vi "Handling Incoming Bytes Tests.vi"(8 "error in (no error)":errorcluster) -> (0 "error out":errorcluster)   [LabVIEW 2013]
uses:
  source/Control Packets/ControlPacket/Control Packet Type -- enum.ctl
  source/Control Packets/CONNACK/Connect Return Code -- enum.ctl
  source/Control Packets/SUBSCRIBE/Topic Subscription -- cluster.ctl
  source/Control Packets/ControlPacket/QualityOfService -- enum.ctl
  source/Control Packets/SUBACK/Subscription Success Code.ctl
  source/Control Packets/CONNECT/ConnectPayload -- cluster.ctl
  source/Control Packets/ControlPacket/ControlPacket.lvclass
  source/Control Packets/CONNECT/CONNECT.lvclass
  source/Control Packets/CONNACK/CONNACK.lvclass
  source/Control Packets/PINGREQ/PINGREQ.lvclass
  source/Control Packets/PINGRESP/PINGRESP.lvclass
  source/Control Packets/PUBACK/PUBACK.lvclass
  source/Control Packets/PUBCOMP/PUBCOMP.lvclass
  source/Control Packets/PUBLISH/PUBLISH.lvclass
  source/Control Packets/PUBREC/PUBREC.lvclass
  source/Control Packets/PUBREL/PUBREL.lvclass
  source/Control Packets/SUBACK/SUBACK.lvclass
  source/Control Packets/SUBSCRIBE/SUBSCRIBE.lvclass
  source/Control Packets/UNSUBACK/UNSUBACK.lvclass
  source/Control Packets/UNSUBSCRIBE/UNSUBSCRIBE.lvclass
  source/Control Packets/DISCONNECT/DISCONNECT.lvclass
  <vilib>/addons/_JKI Toolkits/Caraya/classes/Test/Test.lvclass
panel:
  out "Packets Encoded":T1[](array[typedef])
  out "Packets decoded":T1[](array[typedef])
  out "Split message in single byte transmissions":bool
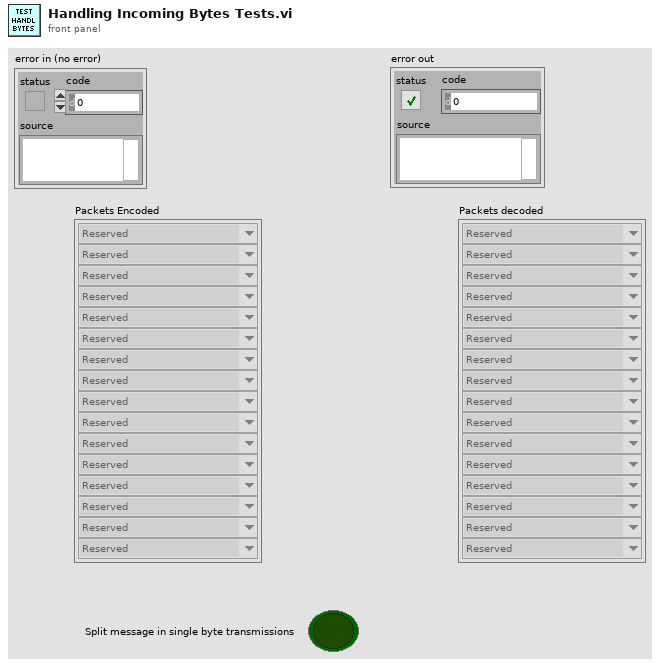
[diagram p1: front panel]
types:
  T1 = typedef "MQTT_Control_Packets.lvlib/ControlPacket.lvclass/Control Packet Type -- enum.ctl" = enum16{"Reserved", "CONNECT", "CONNACK", "PUBLISH", "PUBACK", "PUBREC", "PUBREL", "PUBCOMP", "SUBSCRIBE", "SUBACK", "UNSUBSCRIBE", "UNSUBACK", "PINGREQ", "PINGRESP", "DISCONNECT", "AUTH"}
  T2 = typedef "MQTT_Control_Packets.lvlib/CONNECT.lvclass/ConnectPayload -- cluster.ctl" = cluster{"Will Topic":string, "Will Message":string, "Username":string, "Password":string}
  T3 = typedef "MQTT_Control_Packets.lvlib/SUBACK.lvclass/Subscription Success Code.ctl" = cluster{"Subscription Failure":bool, "QoS":T4}
  T4 = typedef "MQTT_Control_Packets.lvlib/ControlPacket.lvclass/QualityOfService -- enum.ctl" = enum16{"0 (At Most Once)", "1 (At Least Once)", "2 (Exactly Once)"}
  T5 = typedef "MQTT_Control_Packets.lvlib/SUBSCRIBE.lvclass/Topic Subscription -- cluster.ctl" = cluster{"Topic Filter":string, "QoS":T4}
  T6 = typedef "MQTT_Control_Packets.lvlib/CONNACK.lvclass/Connect Return Code -- enum.ctl" = enum16{"Connection accepted", "Unacceptable protocol version", "Identifier Rejected", "Server Unavailable", "Bad Username or Password", "Not Authorized"}
  T7 = cluster{"Control Packet Type":T1, "Bytes Stream":u8[]}
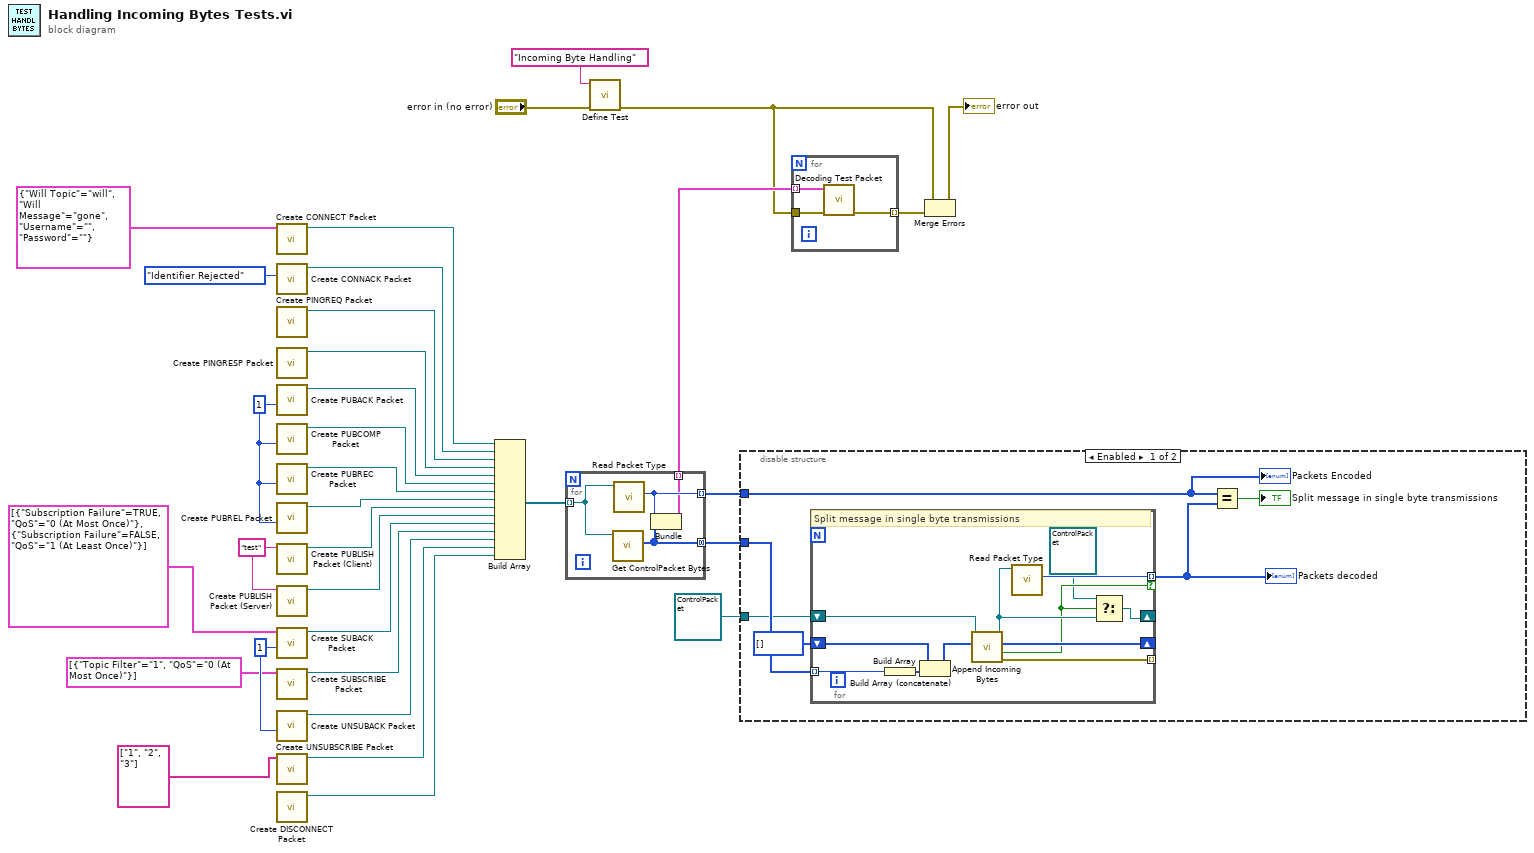
[diagram p0: block diagram]
diagram:
  w19 = u16 1 ("Packet ID")
  w22 = "test" ("Topic Name")
  w24 = u16 1 ("Packet ID")
  n1 = call "Create CONNECT Packet.vi"("Payload"=T2 {"Will Topic"="will", "Will Message"="gone", "Username"="", "Password"=""}) -> ("CONNECT"=w28:refnum<class "CONNECT.lvclass">)  [unwired: 9 in, 1 out]
  n2 = call "Create CONNACK Packet.vi"("Return Code"=Connect_Return_Code_--_enum."Identifier Rejected") -> ("CONNACK"=w32:refnum<class "CONNACK.lvclass">)  [unwired: 9 in, 1 out]
  n3 = call "Create PINGREQ Packet.vi"() -> ("PINGREQ out"=w31:refnum<class "PINGREQ.lvclass">)  [unwired: 10 in, 1 out]
  n4 = call "Create PINGRESP Packet.vi"() -> ("PINGRESP out"=w30:refnum<class "PINGRESP.lvclass">)  [unwired: 10 in, 1 out]
  n5 = call "Create PUBACK Packet.vi"("Packet ID"=w24) -> ("PUBACK out"=w27:refnum<class "PUBACK.lvclass">)  [unwired: 9 in, 1 out]
  n6 = call "Create PUBCOMP Packet.vi"("Packet ID"=w24) -> ("PUBCOMP out"=w26:refnum<class "PUBCOMP.lvclass">)  [unwired: 9 in, 1 out]
  n7 = call "Create PUBREC Packet.vi"("Packet ID"=w24) -> ("PUBREC out"=w25:refnum<class "PUBREC.lvclass">)  [unwired: 9 in, 1 out]
  n8 = call "Create PUBREL Packet.vi"("Packet ID"=w24) -> ("PUBREL out"=w23:refnum<class "PUBREL.lvclass">)  [unwired: 9 in, 1 out]
  n9 = call "Create PUBLISH Packet (Client).vi"("Topic Name"=w22) -> ("PUBLISH"=w21:refnum<class "PUBLISH.lvclass">)  [unwired: 8 in, 2 out]
  n10 = call "Create PUBLISH Packet (Server).vi"("Topic Name"=w22) -> ("PUBLISH"=w20:refnum<class "PUBLISH.lvclass">)  [unwired: 8 in, 2 out]
  n11 = call "Create SUBACK Packet.vi"("Packet ID"=w19, "Return Codes"=T3[] [{"Subscription Failure"=TRUE, "QoS"=enum."0 (At Most Once)"}, {"Subscription Failure"=FALSE, "QoS"=enum."1 (At Least Once)"}]) -> ("SUBACK"=w11:refnum<class "SUBACK.lvclass">)  [unwired: 8 in, 1 out]
  n12 = call "Create SUBSCRIBE Packet.vi"("Topic Subscriptions"=T5[] [{"Topic Filter"="1", "QoS"=enum."0 (At Most Once)"}]) -> ("SUBSCRIBE out"=w12:refnum<class "SUBSCRIBE.lvclass">)  [unwired: 9 in, 1 out]
  n13 = call "Create UNSUBACK Packet.vi"("Packet ID"=w19) -> ("UNSUBACK out"=w13:refnum<class "UNSUBACK.lvclass">)  [unwired: 9 in, 1 out]
  n14 = call "Create UNSUBSCRIBE Packet.vi"("Topic Subscriptions"=string[] ["1", "2", "3"]) -> ("UNSUBSCRIBE out"=w18:refnum<class "UNSUBSCRIBE.lvclass">)  [unwired: 9 in, 1 out]
  n15 = call "Create DISCONNECT Packet.vi"() -> ("DISCONNECT"=w17:refnum<class "DISCONNECT.lvclass">)  [unwired: 10 in, 1 out]
  n16 = Build Array(w28, w32, w31, w30, w27, w26, w25, w23, w21, w20, w11, w12, w13, w18, w17) -> (w29:refnum<class "ControlPacket.lvclass">[])
  n17 = for {
    tunnel: w29 -> [w37] mode=indexing
    tunnel: [w35] -> w9 mode=concatenating
    tunnel: [w36] -> w7 mode=indexing
    tunnel: [w34] -> w8 mode=indexing
    n18 = call "Get ControlPacket Bytes.vi"("ControlPacket"=w37) -> ("Bytes Stream"=w35:u8[])  [unwired: 7 in, 3 out]
    n19 = call "Read Packet Type.vi"("ControlPacket in"=w37) -> ("Control Packet Type"=w36:T1)  [unwired: 9 in, 1 out]
    n20 = Bundle("Control Packet Type"=w36, "Bytes Stream"=w35) -> (w34:T7)  [unwired: 1 in]
  }
  n21 = call <vilib>:"Define Test.vi"("error in (no error)"="error in (no error)", "Label (VI Title)"="Incoming Byte Handling") -> ("error out"=w4:errorcluster)  [unwired: 9 in]
  n22 = disable-structure shown="Enabled" {
    disable-tunnel: w9 -> [w40 _]
    disable-tunnel: w7 -> [w39 _]
    disable-tunnel: refnum<class "ControlPacket.lvclass"> refnum ("ControlPacket") -> [w38 _]
    frame Enabled {
      n23 = for {
        tunnel: w40 -> [w55] mode=indexing
        tunnel: [w54] -> w42 mode=indexing if=w46
        tunnel: [w53] -> _ mode=indexing
        shift-right: [w47] -> _
        shift-left: w38 -> [w45]
        shift-right: [w51] -> _
        shift-left: u8[] [] ("Remaining Packets") -> [w50]
        # "Split message in single byte transmissions"
        n24 = Build Array(w55) -> (w49:u8[])
        n25 = Build Array (concatenate)(w50, w49) -> (w52:u8[])
        n26 = call "Append Incoming Bytes.vi"("Incoming Packets"=w52, "Incomplete ControlPacket"=w45) -> ("error out"=w53:errorcluster, "Complete Packet"=w46:bool, "Remaining Packets"=w51:u8[], "ControlPacket"=w48:refnum<class "ControlPacket.lvclass">)  [unwired: 6 in]
        n27 = call "Read Packet Type.vi"("ControlPacket in"=w48) -> ("Control Packet Type"=w54:T1)  [unwired: 9 in, 1 out]
        n28 = Select(t=refnum<class "ControlPacket.lvclass"> refnum ("ControlPacket"), s=w46, f=w48) -> (s? t:f=w47:refnum<class "ControlPacket.lvclass">)
      }
      "Packets decoded" <- w42
      n29 = Equal?(x=w39, y=w42) -> (x = y?=→"Split message in single byte transmissions":bool)
      "Packets Encoded" <- w39
    }
    frame Disabled {
    }
  }
  n30 = for {
    tunnel: w8 -> [w58] mode=indexing
    tunnel: w4 -> [w57]
    tunnel: [w56] -> w3 mode=indexing
    n31 = call "Decoding Test Packet.vi"("error in (no error)"=w57, "Test Packet Input"=w58) -> ("error out"=w56:errorcluster)  [unwired: 9 in]
  }
  n32 = Merge Errors(w4, w3) -> (→"error out":errorcluster)
